vi "Tank Situation.vi"(7 "Water":i16, 8 "error in":errorcluster, 9 "Milk":i16, 10 "Coffee":i16) -> (0 "error out":errorcluster)   [LabVIEW 2024, in "Tank.lvlib"]
doc: "Send tank status to other modules.\n_____\nCreated using DQMH Event Scripter 7.0.1.1316."
uses:
  Tank.lvlib
  Tank Situation Argument--cluster.ctl
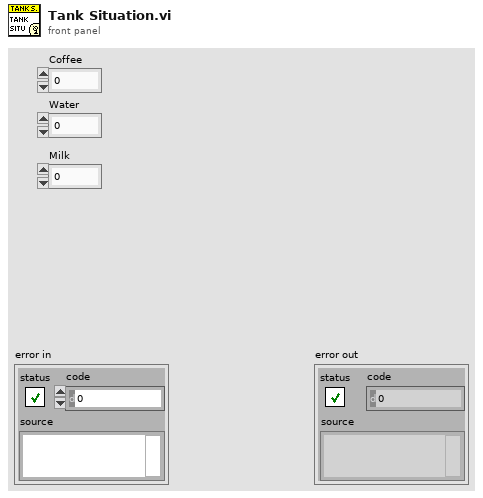
[diagram p1: front panel]
types:
  T1 = typedef "Tank.lvlib/Tank Situation Argument--cluster.ctl" = cluster{"Coffee":i16, "Milk":i16, "Water":i16}
  T2 = typedef "Tank.lvlib/Broadcast Events--cluster.ctl" = cluster{"Module Did Init":refnum<user-event>, "Status Updated":refnum<user-event>, "Error Reported":refnum<user-event>, "Module Did Stop":refnum<user-event>, "Update Module Execution Status":refnum<user-event>, "Tank Situation":refnum<user-event>}
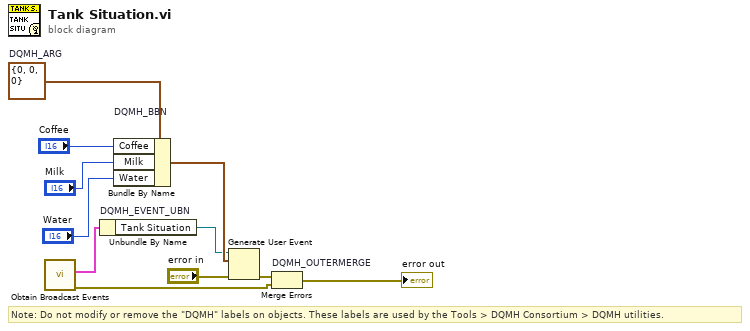
[diagram p0: block diagram]
diagram:
  w6 = T1 {"Coffee"=0, "Milk"=0, "Water"=0}  # DQMH_ARG
  # "Note: Do not modify or remove the \"DQMH\" labels on objects. These labels are used by the Tools > DQMH Consortium > DQMH utilities."
  n1 = call "Obtain Broadcast Events.vi"() -> ("error out"=w2:errorcluster, "Tank Broadcast Events"=w1:T2)  [unwired: 10 in]
  n2 = Unbundle By Name "DQMH_EVENT_UBN"(w1) -> ("Tank Situation"=w8:refnum<user-event>)
  n3 = Bundle By Name "DQMH_BBN"(cluster=w6, "Coffee"="Coffee", "Milk"="Milk", "Water"="Water") -> (w9:T1)
  n4 = Generate User Event(user event=w8, event data cluster=w9, error in="error in") -> (error out=w7:errorcluster)  [unwired: 1 in, 1 out]
  n5 = Merge Errors "DQMH_OUTERMERGE"(w7, w2) -> (→"error out":errorcluster)
